vi "Command_Acquire_Hatch.vi"(2 "Startup":bool) -> (1 "Disc":T1, 3 "Reint":bool, 4 "Completed":bool, 5 "Press":T1)   [LabVIEW 2018]
uses:
  <vilib>/Rock Robotics/WPI/Solenoid/WPI_SolenoidValue.ctl
  Autonomous Utilities/Command_Execution_State.ctl
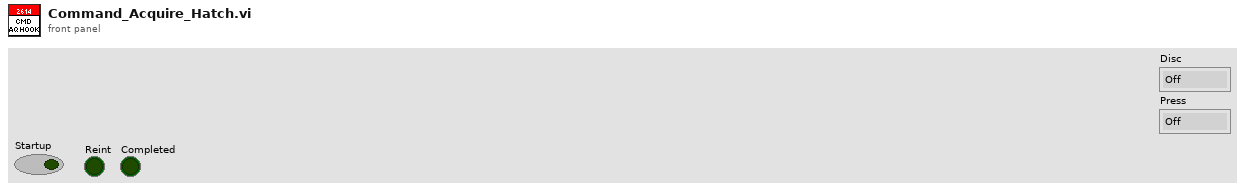
[diagram p1: front panel]
types:
  T1 = typedef "WPI_SolenoidValue.ctl" = enum16{"Off", "On", "Forward", "Reverse"}
  T2 = typedef "Command_Execution_State.ctl" = enum16{"Initialize", "Execute", "Finish"}
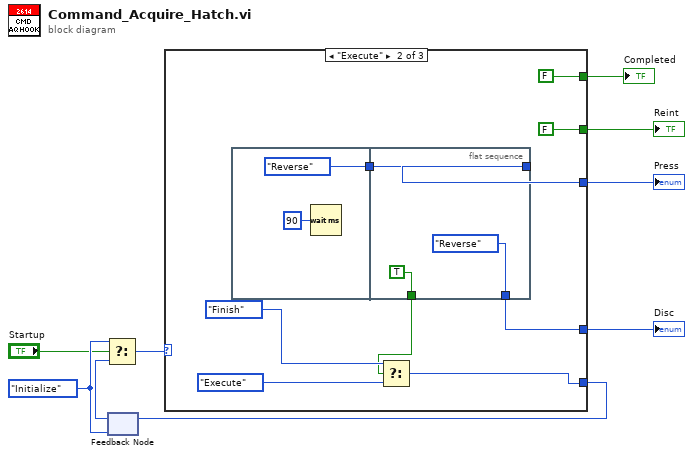
[diagram p0: block diagram]
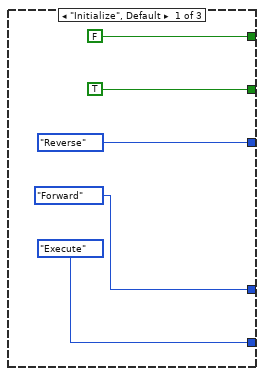
[diagram p2: hidden frame]
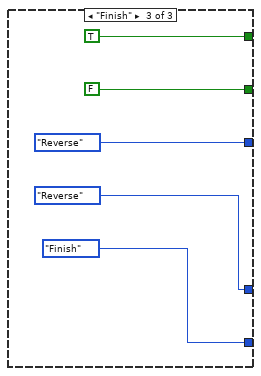
[diagram p3: hidden frame]
diagram:
  w6 = Command_Execution_State."Initialize" ("Play State")
  n1 = feedback #1(w6) -> (w7:T2)
  n2 = Select(t=w6, s="Startup", f=w7) -> (s? t:f=w9:T2)
  n3 = case shown="\"Execute\"" w9 {
    tunnel: [Command_Execution_State."Execute" ("Play State") w19 Command_Execution_State."Finish" ("Play State")] -> w8
    tunnel: [FALSE FALSE TRUE] -> w3
    tunnel: [TRUE FALSE FALSE] -> w4
    tunnel: [WPI_SolenoidValue."Reverse" ("y") w18 WPI_SolenoidValue."Reverse" ("y")] -> w2
    tunnel: [WPI_SolenoidValue."Forward" ("y") w15 WPI_SolenoidValue."Reverse" ("y")] -> w1
    frame "Initialize", Default {
    }
    frame "Execute" {
      n4 = flat-sequence {
        tunnel: [WPI_SolenoidValue."Reverse" ("y")] -> w17
        tunnel: [w28] -> w18
        tunnel: w17 -> [w28]
        tunnel: [TRUE ("s")] -> w16
        tunnel: [WPI_SolenoidValue."Reverse" ("y")] -> w15
        frame #0 {
          n5 = Wait (ms)(milliseconds to wait=u32 90) -> ()  [unwired: 1 out]
        }
        frame #1 {
        }
      }
      n6 = Select(t=Command_Execution_State."Finish" ("Play State"), s=w16, f=Command_Execution_State."Execute" ("Play State")) -> (s? t:f=w19:T2)
    }
    frame "Finish" {
    }
  }
  "Reint" <- w4
  "Completed" <- w3
  "Disc" <- w1
  "Press" <- w2
  n7 = feedback-in #1(w8) -> ()
